vi "ls_data.vi"(7 "LabVIEW Web Service Request":refnum<class "Web Request.lvclass">) -> ()   [LabVIEW 2019]
uses:
  <vilib>/wsapi/Web Request.lvclass
panel:
  # "Use the Web Service Request input terminal to call the VIs on the Web Services palette. Do not remove it from the connector pane unless you don't need access to the palette."
  # "Each additional control wired to the connector pane will be available as an input in the URL. To include an indicator in terminal-mode output (the default setting), it must also be wired to the connector pane."
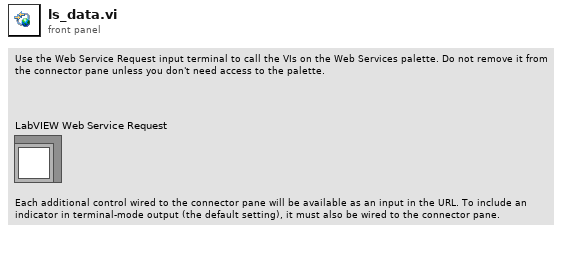
[diagram p1: front panel]
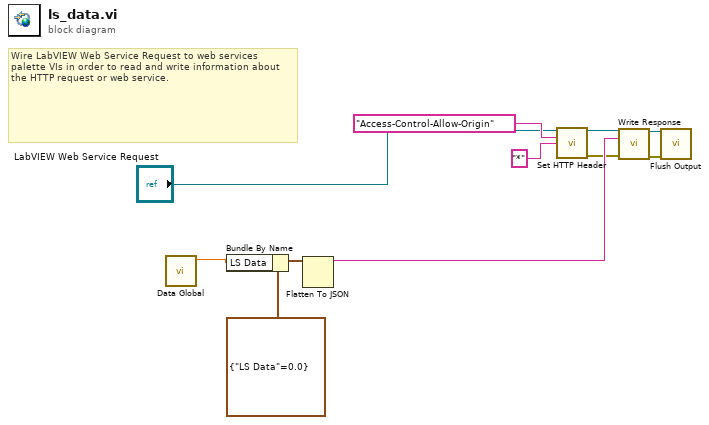
[diagram p0: block diagram]
diagram:
  # "Wire LabVIEW Web Service Request to web services palette VIs in order to read and write information about the HTTP request or web service."
  n1 = call "Data Global.vi"() -> ("Data OUT"=w1:dbl)  [unwired: 11 in]
  n2 = Bundle By Name(cluster=cluster{"LS Data":dbl} {"LS Data"=0.0}, "LS Data"=w1) -> (w2:cluster{"LS Data":dbl})
  n3 = Flatten To JSON(anything=w2) -> (JSON string=w5:string)  [unwired: 2 in, 1 out]
  n4 = call <vilib>:"Set HTTP Header.vi"("LabVIEW Web Service Request"="LabVIEW Web Service Request", "header"="Access-Control-Allow-Origin", "header value"="*") -> ("LabVIEW Web Service Request out"=w6:refnum<class "Web Request.lvclass">, "error out"=w4:errorcluster)  [unwired: 11 in]
  n5 = call <vilib>:"Write Response.vi"("LabVIEW Web Service Request"=w6, "response string"=w5, "error in (no error)"=w4) -> ("LabVIEW Web Service Request out"=w7:refnum<class "Web Request.lvclass">, "error out"=w8:errorcluster)  [unwired: 11 in]
  n6 = call <vilib>:"Flush Output.vi"("LabVIEW Web Service Request"=w7, "error in (no error)"=w8) -> ()  [unwired: 12 in, 2 out]
